vi "positionManager.vi"(5 "Display":u16=1, 6 "just calculate":bool, 9 "Cluster":T1={"Xoffset"=0.0, "Yoffset in"=0.0, "X position in"=-2.9872204472843453, "Y position in"=0.9349593495934956, "Fine X position"=-0.8785942492012779, "Fine Y position"=2.6518218623481786, "Reverse X"=0, "Reverse Y"=0, "XYswap"=0} {"XYswap" items=["swap", "direct"]; "Reverse Y" items=["direct", "reverse"]; "Reverse X" items=["direct", "reverse"]; "Fine Y position" scale=0.0..10.0; "Fine X position" scale=0.0..10.0; "Y position in" scale=0.0..10.0; "X position in" scale=0.0..10.0}) -> (0 "Y position out":i32=60, 1 "X position out":i32=-54, 3 "output cluster":cluster{i32, i32}={-54, 60})   [LabVIEW 2023]
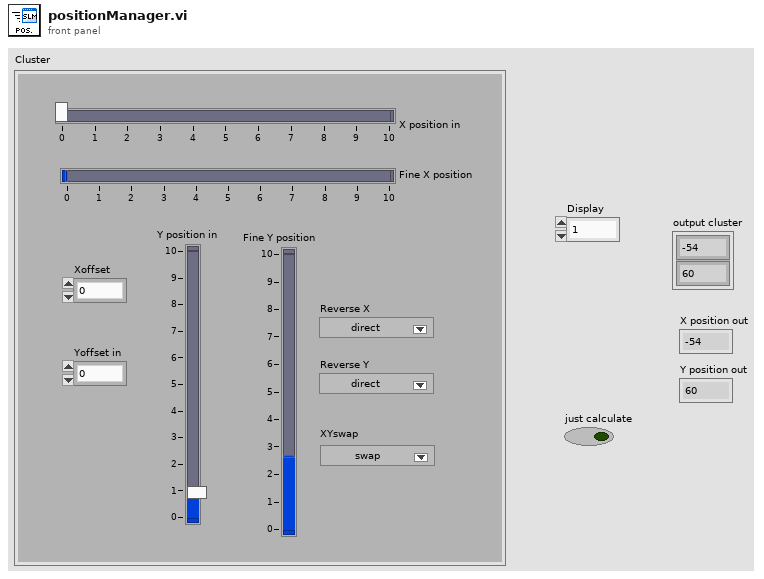
[diagram p1: front panel]
types:
  T1 = cluster{"Xoffset":dbl, "Yoffset in":dbl, "X position in":dbl, "Y position in":dbl, "Fine X position":dbl, "Fine Y position":dbl, "Reverse X":u16, "Reverse Y":u16, "XYswap":u16}
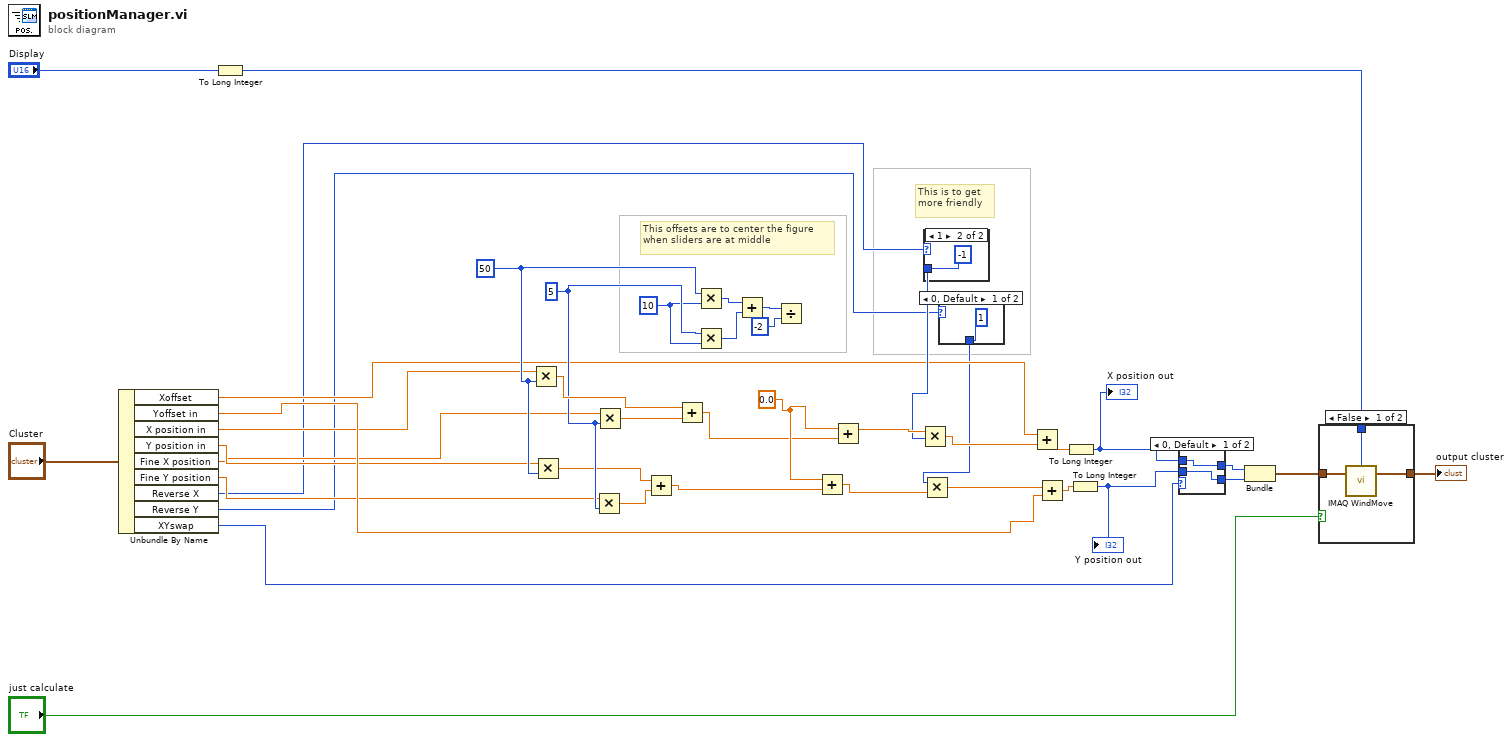
[diagram p0: block diagram]
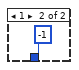
[diagram p4: hidden frame]
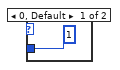
[diagram p5: hidden frame]
diagram:
  w41 = 0.0 ("x")
  w26 = 10 ("y")
  w27 = 5
  w25 = 50
  # "This is to get more friendly"
  # "This offsets are to center the figure when sliders are at middle"
  n1 = Unbundle By Name("Cluster") -> ("Xoffset"=w21:dbl, "Yoffset in"=w20:dbl, "X position in"=w19:dbl, "Y position in"=w18:dbl, "Fine X position"=w17:dbl, "Fine Y position"=w16:dbl, "Reverse X"=w10:u16, "Reverse Y"=w9:u16, "XYswap"=w6:u16)
  n2 = To Long Integer(number="Display") -> (32bit integer=w4:i32)
  n3 = Multiply(x=w19, y=w25) -> (x*y=w32:dbl)
  n4 = Multiply(x=w18, y=w25) -> (x*y=w23:dbl)
  n5 = Multiply(x=w16, y=w27) -> (x*y=w24:dbl)
  n6 = Multiply(x=w17, y=w27) -> (x*y=w33:dbl)
  n7 = Add(x=w23, y=w24) -> (x+y=w35:dbl)
  n8 = Add(x=w32, y=w33) -> (x+y=w34:dbl)
  n9 = Multiply(x=w25, y=w26) -> (x*y=w28:i32)
  n10 = Multiply(x=w27, y=w26) -> (x*y=w29:i32)
  n11 = Add(x=w28, y=w29) -> (x+y=w30:i32)
  n12 = Divide(x=w30, y=-2) -> ()  [unwired: 1 out]
  n13 = Add(x=w41, y=w35) -> (x+y=w38:dbl)
  n14 = Add(x=w41, y=w34) -> (x+y=w37:dbl)
  n15 = case shown="1" w10 {
    tunnel: [1 ("y") -1 ("y")] -> w36
    frame 0, Default {
    }
    frame 1 {
    }
  }
  n16 = Multiply(x=w37, y=w36) -> (x*y=w39:dbl)
  n17 = case shown="0, Default" w9 {
    tunnel: [1 ("y") -1 ("y")] -> w11
    frame 0, Default {
    }
    frame 1 {
    }
  }
  n18 = Multiply(x=w11, y=w38) -> (x*y=w40:dbl)
  n19 = Add(x=w21, y=w39) -> (x+y=w15:dbl)
  n20 = Add(x=w40, y=w20) -> (x+y=w14:dbl)
  n21 = To Long Integer(number=w15) -> (32bit integer=w2:i32)
  "X position out" <- w2
  n22 = To Long Integer(number=w14) -> (32bit integer=w1:i32)
  "Y position out" <- w1
  n23 = case shown="0, Default" w6 {
    tunnel: [w46 w49] -> w8
    tunnel: w2 -> [w47 w49]
    tunnel: [w47 w48] -> w7
    tunnel: w1 -> [w46 w48]
    frame 0, Default {
    }
    frame 1 {
    }
  }
  n24 = Bundle(w7, w8) -> (w13:cluster{i32, i32})  [unwired: 1 in]
  n25 = case shown="False" "just calculate" {
    tunnel: w13 -> [w52 w53]
    tunnel: [w51 w53] -> w12
    tunnel: w4 -> [w50 _]
    frame False {
      n26 = call "IMAQ WindMove"("Window Number (0...15)"=w50, "Coordinates (screen)"=w52) -> ("Coordinates (screen)"=w51:cluster{"X Position":i32, "Y Position":i32})  [unwired: 3 in, 1 out]
    }
    frame True {
    }
  }
  "output cluster" <- w12
